vi "test CopySmallerDestinationvi.vi"(8 "error in (no error)":errorcluster, 11 "TestCase in":refnum<class "Data Manipulation Tests.lvclass">) -> (0 "error out":errorcluster, 3 "TestCase out":refnum<class "Data Manipulation Tests.lvclass">)   [LabVIEW 2017, in "Pointer Tests.lvlib" / "Data Manipulation Tests.lvclass"]
uses:
  Data Manipulation Tests.lvclass
  Source/Classes/Pointer/Public/New/New (4B).vi
  Source/Classes/Pointer/Public/Write/Write (1D I32).vi
  Source/Classes/Pointer/Public/New/New (2B).vi
  Source/Classes/Pointer/Public/Read/Read (1D I32).vi
  <vilib>/addons/_JKI Toolkits/VI Tester/TestCase.llb/TestCase.lvclass
  Source/Classes/Pointer/Pointer.lvclass
  C:/Program Files (x86)/National Instruments/LabVIEW 2017/vi.lib/addons/_JKI Toolkits/VI Tester/TestCase.llb/TestCase.lvclass
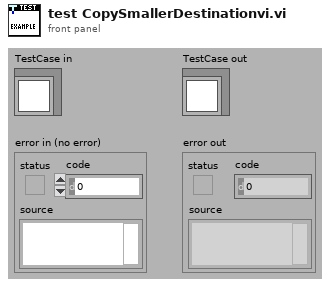
[diagram p1: front panel]
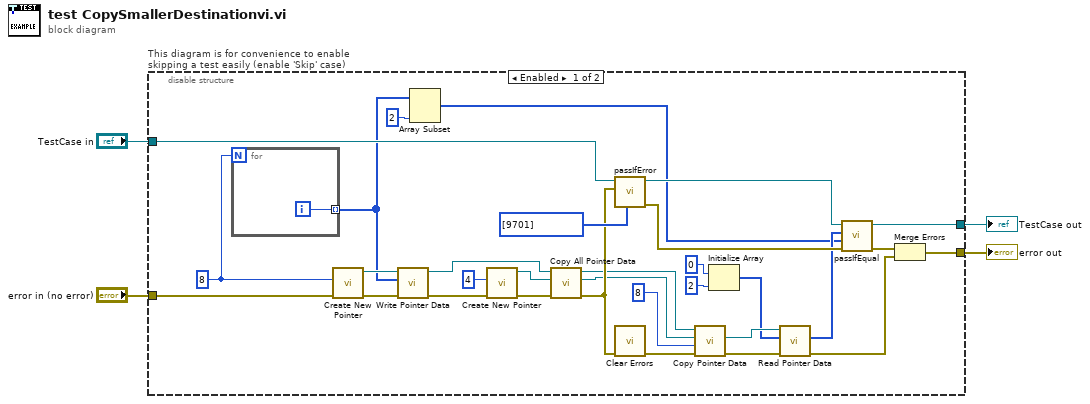
[diagram p0: block diagram]
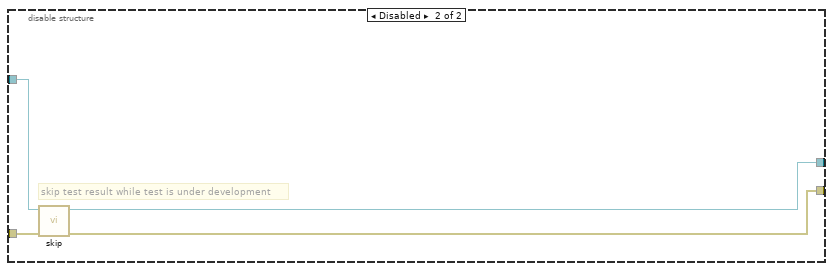
[diagram p2: hidden frame]
diagram:
  n1 = disable-structure "This diagram is for convenience to enable skipping a test easily (enable 'Skip' case)" shown="Enabled" {
    disable-tunnel: "TestCase in" -> [w31 w40]
    disable-tunnel: [w13 w38] -> w1
    disable-tunnel: [w26 w39] -> w3
    disable-tunnel: "error in (no error)" -> [w30 w37]
    frame Enabled {
      w17 = u64 8 ("count (1)")
      n2 = for {
        N: w17 -> [_]
        tunnel: [w36] -> w8 mode=indexing
        i -> [w36]
      }
      n3 = call-poly "Create New Pointer.vi"("error in (no error)"=w30, "count (1)"=w17) -> ("error out"=w29:errorcluster, "Pointer"=w35:refnum<class "Pointer.lvclass">)  [unwired: 8 in]
      n4 = call-poly "Write Pointer Data.vi"("error in (no error)"=w29, "buffer in"=w8, "Pointer in"=w35) -> ("error out"=w28:errorcluster, "Pointer out"=w34:refnum<class "Pointer.lvclass">)  [unwired: 5 in, 2 out]
      n5 = Array Subset(array=w8, length=2) -> (w6:i32[])  [unwired: 1 in]
      n6 = call-poly "Create New Pointer.vi"("error in (no error)"=w28, "count (1)"=u64 4) -> ("error out"=w27:errorcluster, "Pointer"=w33:refnum<class "Pointer.lvclass">)  [unwired: 8 in]
      n7 = call "Copy All Pointer Data.vi"("error in (no error)"=w27, "dst Pointer in"=w33, "src Pointer in"=w34) -> ("error out"=w24:errorcluster, "dst Pointer out"=w9:refnum<class "Pointer.lvclass">, "src Pointer out"=w21:refnum<class "Pointer.lvclass">)  [unwired: 6 in]
      n8 = call-dynamic "passIfError.vi"("passing error codes (default = any error code)"=i32[] [9701], "error"=w24, "TestCase in"=w31) -> ("error out"=w32:errorcluster, "TestCase out"=w14:refnum<class "Data Manipulation Tests.lvclass">)  [unwired: 7 in]
      n9 = call <vilib>:"Clear Errors.vi"("error in (no error)"=w24) -> ("error out"=w23:errorcluster)  [unwired: 5 in, 1 out]
      n10 = call "Copy Pointer Data.vi"("error in (no error)"=w23, "bytes to copy"=u64 8, "dst Pointer in"=w9, "src Pointer in"=w21) -> ("error out"=w22:errorcluster, "dst Pointer out"=w19:refnum<class "Pointer.lvclass">)  [unwired: 4 in, 2 out]
      n11 = Initialize Array(0 ("Numeric"), 2 ("dimension size")) -> (w16:i32[])
      n12 = call-poly "Read Pointer Data.vi"("error in (no error)"=w22, "buffer in"=w16, "Pointer in"=w19) -> ("error out"=w20:errorcluster, "buffer out"=w12:i32[])  [unwired: 5 in, 2 out]
      n13 = call-dynamic "passIfEqual.vi"("error in (no error)"=w32, "y"=w6, "x"=w12, "TestCase in"=w14) -> ("error out"=w15:errorcluster, "TestCase out"=w13:refnum<class "Data Manipulation Tests.lvclass">)  [unwired: 6 in]
      n14 = Merge Errors(w15, w20) -> (w26:errorcluster)
    }
    frame Disabled {
      # "skip test result while test is under development"
      n15 = call <vilib>:"skip.vi"("error in (no error)"=w37, "TestCase in"=w40) -> ("error out"=w39:errorcluster, "TestCase out"=w38:refnum<class "Data Manipulation Tests.lvclass">)  [unwired: 8 in]
    }
  }
  "error out" <- w3
  "TestCase out" <- w1
